vi "initialize AO1 laser task.vi"(8 "error in (no error)":errorcluster, 11 "NI in":refnum<class "NI.lvclass">) -> (0 "error out":errorcluster, 3 "NI out":refnum<class "NI.lvclass">)   [LabVIEW 2021, in "NI.lvlib" / "NI.lvclass"]
uses:
  NI.lvclass
  NI.lvclass/NI.ctl
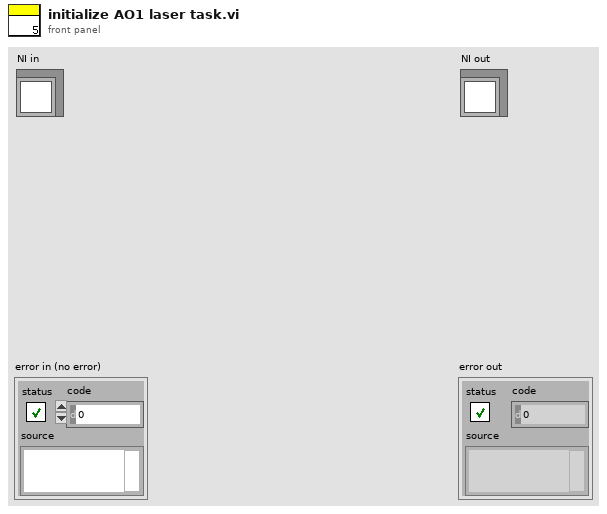
[diagram p1: front panel]
types:
  T1 = typedef "NI.lvlib/NI.lvclass/Channel Connection.ctl" = cluster{"Physical Channel":tag, "Terminal":tag, "StartTrigger":tag, "ClockSource":tag}
  T2 = cluster{"fast clock params":cluster{"fast clock rate":dbl, "off time after trigger":dbl, "cam line read time":dbl, "protect ticks #":dbl}, "AO1 laser Connection":T1, "AO2 zy Connection":T1, "AO3 z Connection (deprecated)":T1, "CO1 mainTrig Connection":T1, "CO2 fastClock Connection":T1, "AI phase Connection":T1}
  T3 = cluster{"fast clock rate":dbl, "off time after trigger":dbl, "cam line read time":dbl, "protect ticks #":dbl}
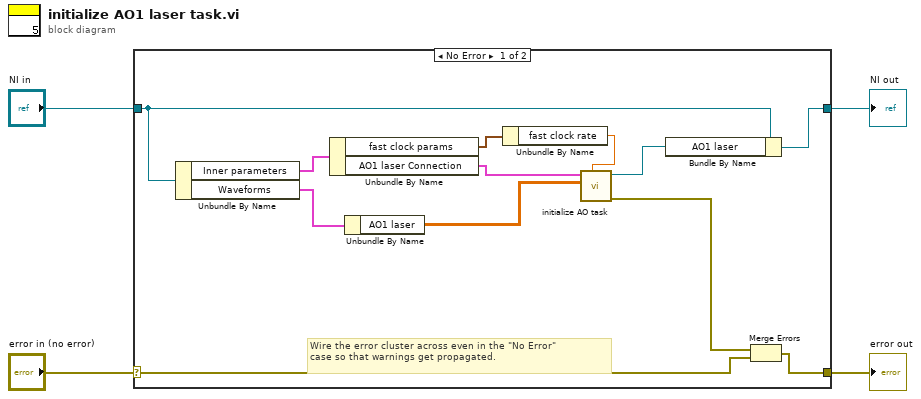
[diagram p0: block diagram]
diagram:
  n1 = case shown="No Error" "error in (no error)" {
    selector: "error in (no error)" -> [w7 w18]
    tunnel: [w6 w18] -> w3
    tunnel: [w9 w17] -> w1
    tunnel: "NI in" -> [w8 w17]
    frame No Error {
      # "Wire the error cluster across even in the \"No Error\"\ncase so that warnings get propagated."
      n2 = Unbundle By Name(w8) -> ("Inner parameters"=w16:T2, "Waveforms"=w15:cluster{"AO1 laser":dbl[][], "AO2 zy":dbl[][]})
      n3 = Unbundle By Name(w16) -> ("fast clock params"=w12:T3, "AO1 laser Connection"=w13:T1)
      n4 = Unbundle By Name(w15) -> ("AO1 laser"=w14:dbl[][])
      n5 = Unbundle By Name(w12) -> ("fast clock rate"=w11:dbl)
      n6 = call "initialize AO task.vi"("rate"=w11, "waveform"=w14, "AO Connection"=w13) -> ("error out"=w5:errorcluster, "task out"=w10:refnum<k21>)  [unwired: 7 in]
      n7 = Bundle By Name(cluster=w8, "AO1 laser"=w10) -> (w9:refnum<class "NI.lvclass">)
      n8 = Merge Errors(w5, w7) -> (w6:errorcluster)
    }
    frame Error {
    }
  }
  "error out" <- w3
  "NI out" <- w1
